vi "Run and wait.vi"(5 "Script":string, 7 "Script Name":string="TSB_Script", 8 "错误输入":errorcluster, 11 "VISA资源名称":refnum<visa-resource-name>) -> (0 "错误输出":errorcluster, 3 "VISA资源名称输出":refnum<visa-resource-name>)   [LabVIEW 2019]
uses:
  Global variable.vi
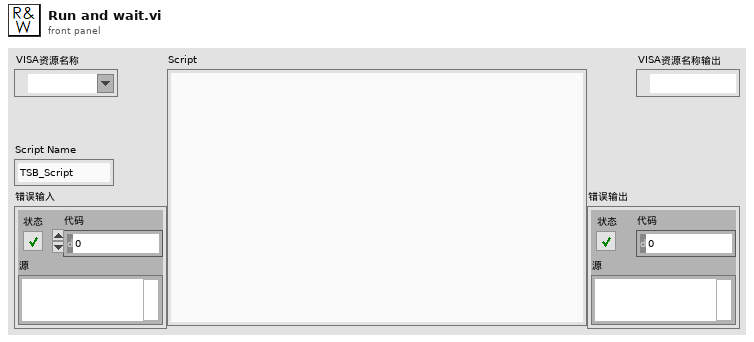
[diagram p1: front panel]
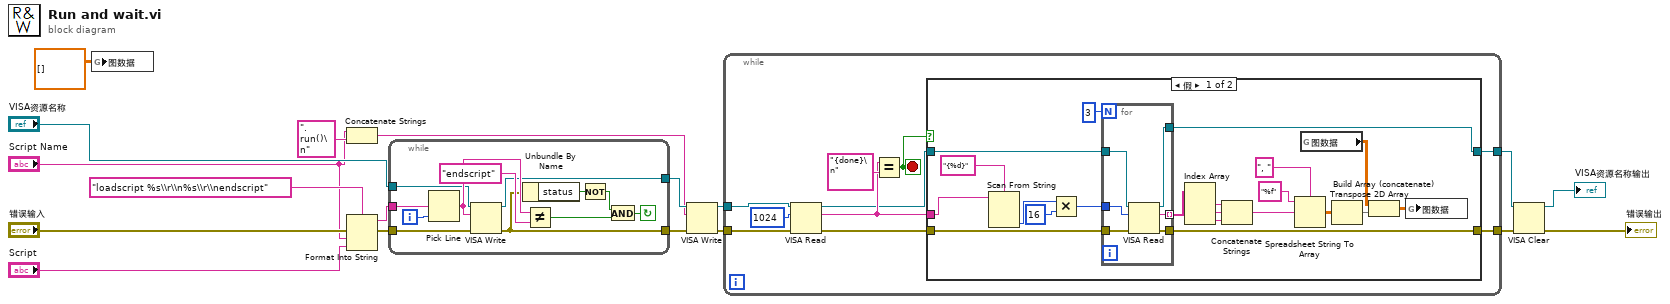
[diagram p0: block diagram]
diagram:
  n1 = global write "Global variable.vi" "图数据"(dbl[][] [] ("图数据")) -> ()
  n2 = Concatenate Strings("Script Name", ".run()\n" ("string")) -> (w8:string)
  n3 = Format Into String(format string="loadscript %s\\r\\n%s\\r\\nendscript", error in="错误输入", "Script Name", "Script") -> (resulting string=w16:string, error out=w13:errorcluster)  [unwired: 1 in]
  n4 = while {
    tunnel: w16 -> [w29]
    tunnel: "VISA资源名称" -> [w22]
    tunnel: w13 -> [w21]
    tunnel: [w20] -> w12
    tunnel: [w19] -> w11
    i -> [w30]
    stop <- w23 continue-if-true
    n5 = Pick Line(multi-line string=w29, line index=w30) -> (output string=w27:string)  [unwired: 1 in]
    n6 = VISA Write(VISA resource name=w22, write buffer=w27, error in (no error)=w21) -> (VISA resource name out=w19:refnum<visa-resource-name>, error out=w20:errorcluster)  [unwired: 1 out]
    n7 = Unbundle By Name(w20) -> ("status"=w26:bool)
    n8 = Not Equal?(x=w27, y="endscript") -> (x != y?=w24:bool)
    n9 = Not(x=w26) -> (.not. x?=w25:bool)
    n10 = And(x=w25, y=w24) -> (x .and. y?=w23:bool)
  }
  n11 = VISA Write(VISA resource name=w11, write buffer=w8, error in (no error)=w12) -> (VISA resource name out=w5:refnum<visa-resource-name>, error out=w4:errorcluster)  [unwired: 1 out]
  n12 = while {
    tunnel: w5 -> [w39]
    tunnel: w4 -> [w38]
    tunnel: [w34] -> w2
    tunnel: [w33] -> w3
    stop <- w31 stop-if-true
    n13 = VISA Read(VISA resource name=w39, byte count=u32 1024 ("字节总数"), error in (no error)=w38) -> (VISA resource name out=w32:refnum<visa-resource-name>, read buffer=w36:string, error out=w35:errorcluster)  [unwired: 1 out]
    n14 = Equal?(x=w36, y="{done}\n") -> (x = y?=w31:bool)
    n15 = case shown="假" w31 {
      tunnel: w36 -> [w61 _]
      tunnel: w35 -> [w59 w68]
      tunnel: [w58 w68] -> w34
      tunnel: [w57 w69] -> w33
      tunnel: w32 -> [w56 w69]
      frame False {
        n16 = Scan From String(format string="{%d}" ("格式字符串"), input string=w61) -> (output 1=w54:i32)  [unwired: 3 in, 3 out]
        n17 = Multiply(x=w54, y=16) -> (x*y=w52:i32)
        n18 = for {
          N: 3 -> [_]
          tunnel: w59 -> [w67]
          tunnel: [w66] -> w58
          tunnel: [w65] -> w57
          tunnel: w56 -> [w64]
          tunnel: w52 -> [w63]
          tunnel: [w62] -> w46 mode=indexing
          n19 = VISA Read(VISA resource name=w64, byte count=w63, error in (no error)=w67) -> (VISA resource name out=w65:refnum<visa-resource-name>, read buffer=w62:string, error out=w66:errorcluster)  [unwired: 1 out]
        }
        n20 = Index Array(array=w46) -> (element #1=w45:string, element #2=w44:string, element #3=w43:string)  [unwired: 3 in]
        n21 = Concatenate Strings(w45, w44, w43) -> (w51:string)
        n22 = Spreadsheet String To Array(delimiter (Tab)=", " ("分隔符(Tab)"), format string="%f" ("格式字符串"), spreadsheet string=w51) -> (array=w48:dbl[][])  [unwired: 1 in]
        n23 = global read "Global variable.vi" "图数据"() -> (w42:dbl[][])
        n24 = Transpose 2D Array(2D array=w48) -> (transposed array=w47:dbl[][])
        n25 = Build Array (concatenate)(w42, w47) -> (w41:dbl[][])
        n26 = global write "Global variable.vi" "图数据"(w41) -> ()
      }
      frame True {
      }
    }
  }
  n27 = VISA Clear(VISA resource name=w3, error in (no error)=w2) -> (VISA resource name out=→"VISA资源名称输出":refnum<visa-resource-name>, error out=→"错误输出":errorcluster)
